vi "Close.vi"(8 "error in (no error)":errorcluster, 11 "DeployResource in":refnum<class "Resource.lvclass">) -> (0 "error out":errorcluster, 3 "DeployResource out":refnum<class "Resource.lvclass">)   [LabVIEW 2020, in "PicoG-Core.lvlib" / "Resource.lvclass"]
uses:
  Resource.lvclass
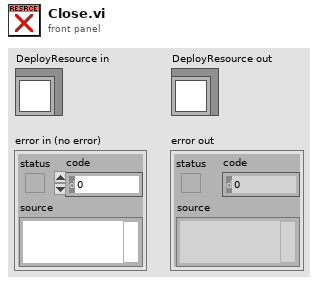
[diagram p1: front panel]
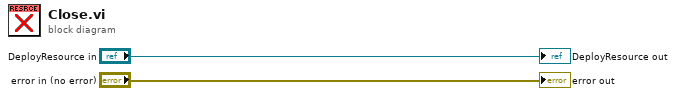
[diagram p0: block diagram]
diagram:
  "error out" <- "error in (no error)"
  "DeployResource out" <- "DeployResource in"
